vi "Radoslaw_Wolnik_3.1_12.vi"() -> ()   [LabVIEW 2012]
uses:
  <vilib>/numeric/Random Number (Range) U64.vi
panel:
  in  "stop":bool
  out "Losowa liczba":i8
  # "Program generuje losowe liczby w zakresie od 0 do 100 co 5s"
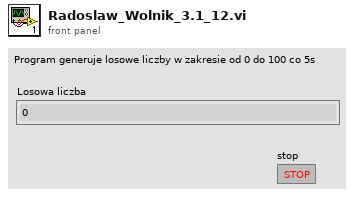
[diagram p1: front panel]
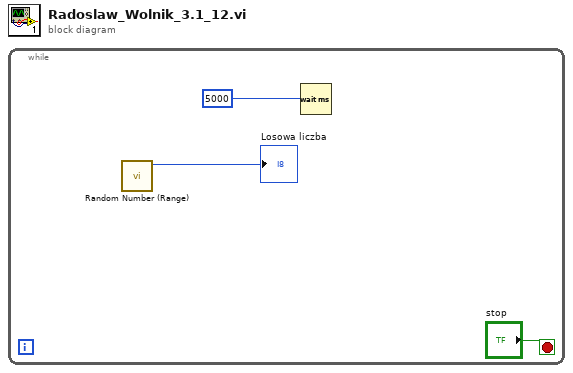
[diagram p0: block diagram]
diagram:
  n1 = while {
    stop <- "stop" stop-if-true
    n2 = call-poly <vilib>:"Random Number (Range).vi"() -> ("number"=→"Losowa liczba":u64)  [unwired: 11 in]
    n3 = Wait (ms)(milliseconds to wait=5000) -> ()  [unwired: 1 out]
  }
